vi "PH_gentec_M-Link.Action check connection.vi"(0 "i ref in":refnum<vi>, 5 "error in":errorcluster) -> (14 "i ref out":refnum<vi>, 19 "error out":errorcluster)   [LabVIEW 2014, in "PH_gentec_M-Link.lvlib"]
uses:
  PH_gentec_M-Link.lvlib
  PH_Powermeter_BaseClass/PH_Powermeter_BaseClass.State.ctl
  non_GPL/instr.lib/gentec-M-LINK/gentec-M-Link - Driver.lvlib
  PH_Powermeter_BaseClass/PH_Powermeter_BaseClass.lvlib
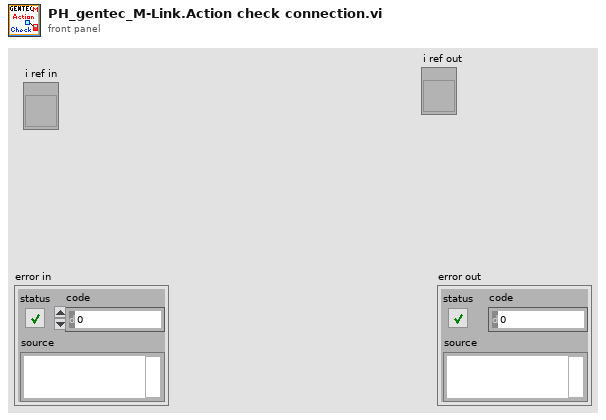
[diagram p1: front panel]
types:
  T1 = typedef "PH_Powermeter_BaseClass.lvlib/PH_Powermeter_BaseClass.State.ctl" = enum32{"off", "operating", "opened", "checked", "connected", "Sets to change", "running"}
  T2 = typedef "PH_Powermeter_BaseClass.lvlib/PH_Powermeter_BaseClass.i attribute.ctl" = cluster{"GUI References":T3, "Connection":T4, "Head Attributes":T5, "VISA resource":refnum<visa-resource-name>, "Energy":T6, "Service ID Energy":i32, "Wanted Settings":T7, "Current Settings":T7}
  T3 = typedef "PH_Powermeter_BaseClass.lvlib/PH_Powermeter_BaseClass.GUI Refs.ctl" = cluster{"Head Attributes":refnum<vi>, "Energy":refnum<vi>, "Connection":refnum<vi>, "VISA Resource":refnum<vi>, "Energy evolution":refnum<vi>, "Scaling Factor":refnum<vi>, "Range":refnum<vi>, "Wavelength":refnum<vi>, "Trigger Level":refnum<vi>, "Wanted Settings":refnum<vi>, "Current Settings":refnum<vi>}
  T4 = typedef "PH_Powermeter_BaseClass.lvlib/PH_Powermeter_BaseClass.Connection.ctl" = cluster{"failed checks":i8, "Timeout":bool, "Data read":string, "Failure":bool, "Error":bool, "State":T1}
  T5 = typedef "PH_Powermeter_BaseClass.lvlib/PH_Powermeter_BaseClass.Head Attributes.ctl" = cluster{"Instrument Type":string, "Head Version":string, "Head Name":string, "Serial Number":string, "Firmware":string, "Sensor Type":string, "MinimumRange":u32, "Maximum Range":u32, "Min Wavelength":i32, "Max Wavelength":i32}
  T6 = typedef "PH_Powermeter_BaseClass.lvlib/PH_Powermeter_BaseClass.Energy.ctl" = cluster{"current Value":dbl, "unscaled":dbl, "Scaling Factor":dbl}
  T7 = typedef "PH_Powermeter_BaseClass.lvlib/PH_gentec_BaseClass.Head Settings.ctl" = cluster{"Trigger Level":dbl, "Wavelength":u32, "Range":u32}
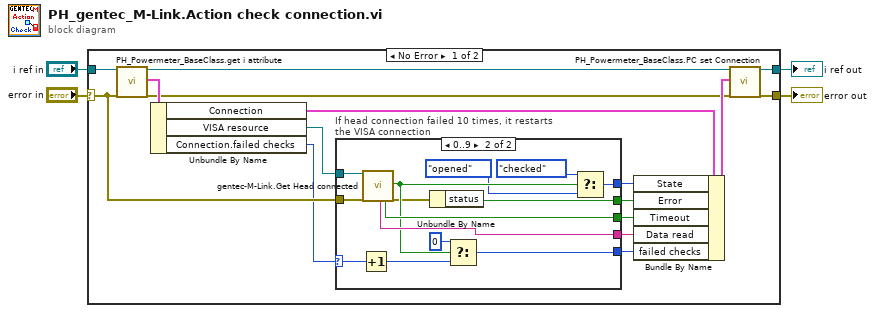
[diagram p0: block diagram]
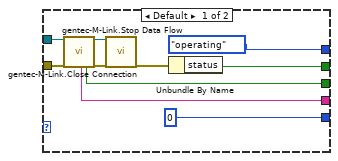
[diagram p2: hidden frame]
diagram:
  n1 = case shown="No Error" "error in" {
    selector: "error in" -> [w15 w46]
    tunnel: "i ref in" -> [w12 w45]
    tunnel: [w8 w45] -> w1
    tunnel: [w7 w46] -> w2
    frame No Error {
      n2 = call "PH_Powermeter_BaseClass.get i attribute.vi"("i ref in"=w12, "error in (no error)"=w15) -> ("i ref out"=w9:refnum<vi>, "i attribute"=w14:T2, "error out"=w6:errorcluster)  [unwired: 15 in]
      n3 = Unbundle By Name(w14) -> ("Connection"=w5:T4, "VISA resource"=w13:refnum<visa-resource-name>, "Connection.failed checks"=w11:i8)
      n4 = case "If head connection failed 10 times, it restarts the VISA connection" shown="0..9" w11 {
        selector: w11 -> [_ w41]
        tunnel: w13 -> [w30 w44]
        tunnel: w15 -> [w29 w40]
        tunnel: [w28 w39] -> w17
        tunnel: [w27 w38] -> w18
        tunnel: [w26 w37] -> w19
        tunnel: [i8 0 ("Connection.failed checks") w36] -> w20
        tunnel: [PH_Powermeter_BaseClass.State."operating" ("State") w33] -> w16
        frame Default {
          n5 = call "gentec-M-Link.Stop Data Flow.vi"("VISA resource In"=w30, "error in (no error)"=w29) -> ("Data Read"=w26:string, "Read Timeout"=w27:bool, "VISA resource Out"=w21:refnum<visa-resource-name>, "error out"=w23:errorcluster)  [unwired: 13 in, 1 out]
          n6 = call "gentec-M-Link.Close Connection.vi"("VISA resource In"=w21, "error in (no error)"=w23) -> ("error out"=w22:errorcluster)  [unwired: 17 in]
          n7 = Unbundle By Name(w22) -> ("status"=w28:bool)
        }
        frame 0..9 {
          n8 = Increment(x=w41) -> (x+1=w43:i8)
          n9 = call "gentec-M-Link.Get Head connected.vi"("VISA resource In"=w44, "error in (no error)"=w40) -> ("Data Read"=w37:string, "Read Timeout"=w38:bool, "Head connected?"=w35:bool, "error out"=w31:errorcluster)  [unwired: 13 in, 1 out]
          n10 = Unbundle By Name(w31) -> ("status"=w39:bool)
          n11 = Select(t=i8 0, s=w35, f=w43) -> (s? t:f=w36:i8)
          n12 = Select(t=PH_Powermeter_BaseClass.State."checked" ("State"), s=w35, f=PH_Powermeter_BaseClass.State."opened" ("State")) -> (s? t:f=w33:T1)
        }
      }
      n13 = Bundle By Name(cluster=w5, "State"=w16, "Error"=w17, "Timeout"=w18, "Data read"=w19, "failed checks"=w20) -> (w10:T4)
      n14 = call "PH_Powermeter_BaseClass.PC set Connection.vi"("VI in"=w9, "Connection"=w10, "error in (no error)"=w6) -> ("VI out"=w8:refnum<vi>, "error out"=w7:errorcluster)  [unwired: 15 in]
    }
    frame Error {
    }
  }
  "error out" <- w2
  "i ref out" <- w1
